vi "Get Window RefNum.vi"(6 "error in (no error)":errorcluster, 9 "window name (\"\")":string) -> (0 "error out":errorcluster, 3 "window refnum (NaWR)":T1)   [LabVIEW 2018]
doc: "This VI will use the FindWindow API function to retrieve a window refnum for the window identified by window name. 'window name' is the text appearing in the title bar of a window. If the window cannot be found, the window refnum out will be 'Not a Window Refnum', and an error will occur."
uses:
  Window Refnum.ctl
  user32.dll
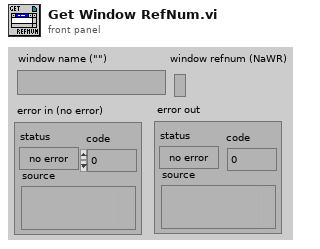
[diagram p1: front panel]
types:
  T1 = typedef "Window Refnum.ctl" = refnum<k1>
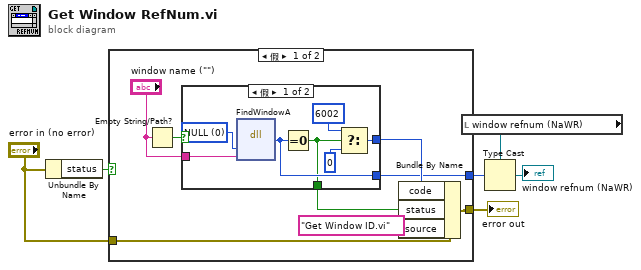
[diagram p0: block diagram]
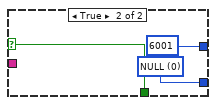
[diagram p2: hidden frame]
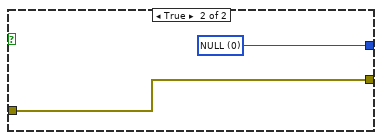
[diagram p3: hidden frame]
diagram:
  n1 = Unbundle By Name("error in (no error)") -> ("status"=w6:bool)
  n2 = case shown="假" w6 {
    tunnel: "error in (no error)" -> [w11 w25]
    tunnel: [w10 w25] -> w4
    tunnel: [w9 w26] -> w3
    frame False {
      n3 = Empty String/Path?(string/path="window name (\"\")") -> (empty?=w8:bool)
      n4 = case shown="假" w8 {
        selector: w8 -> [_ w22]
        tunnel: [w21 w23] -> w9
        tunnel: [w20 w22] -> w13
        tunnel: [w19 6001] -> w14
        tunnel: "window name (\"\")" -> [w15 _]
        frame False {
          w16 = 0 items=["NULL"]
          n5 = dll-call lib="user32.dll" fn="FindWindowA" label="FindWindow"("lpszClassName"=w16, "lpszWindowName"=w15) -> ("hWnd"=w21:u32)  [unwired: 5 in, 2 out]
          n6 = Equal To 0?(x=w21) -> (x = 0?=w20:bool)
          n7 = Select(t=6002, s=w20, f=0) -> (s? t:f=w19:i32)
        }
        frame True {
          w23 = u16 0 items=["NULL"]
        }
      }
      n8 = Bundle By Name(cluster=w11, "code"=w14, "status"=w13, "source"="Get Window ID.vi") -> (w10:errorcluster)
    }
    frame True {
      w26 = u16 0 items=["NULL"]
    }
  }
  "error out" <- w4
  n9 = local read "window refnum (NaWR)"() -> (w1:T1)
  n10 = Type Cast(type=w1, x=w3) -> (*(type *) &x=→"window refnum (NaWR)":T1)
